vi "90 deg probe pitch correction.vi"(3 "az":dbl, 4 "ay":dbl, 5 "ax":dbl) -> (0 "az'":dbl, 1 "ay'":dbl, 2 "ax'":dbl)   [LabVIEW 2020]
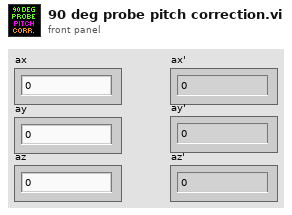
[diagram p1: front panel]
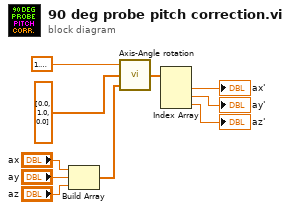
[diagram p0: block diagram]
diagram:
  n1 = Build Array("ax", "ay", "az") -> (w7:dbl[])
  n2 = call "Axis-Angle rotation.vi"("Input vector3"=w7, "Rotation axis (UNIT vector3)"=dbl[] [0.0, 1.0, 0.0], "Rotation angle (rad)"=1.5707963267948966) -> ("Output vector3"=w5:dbl[])
  n3 = Index Array(array=w5) -> (element #1=→"ax'":dbl, element #2=→"ay'":dbl, element #3=→"az'":dbl)  [unwired: 3 in]
